vi "Main Interface.vi"() -> ()   [LabVIEW 2013]
panel:
  in  "Current Task":string
  out "Current Progress":u8(slide) scale=0.0..100.0
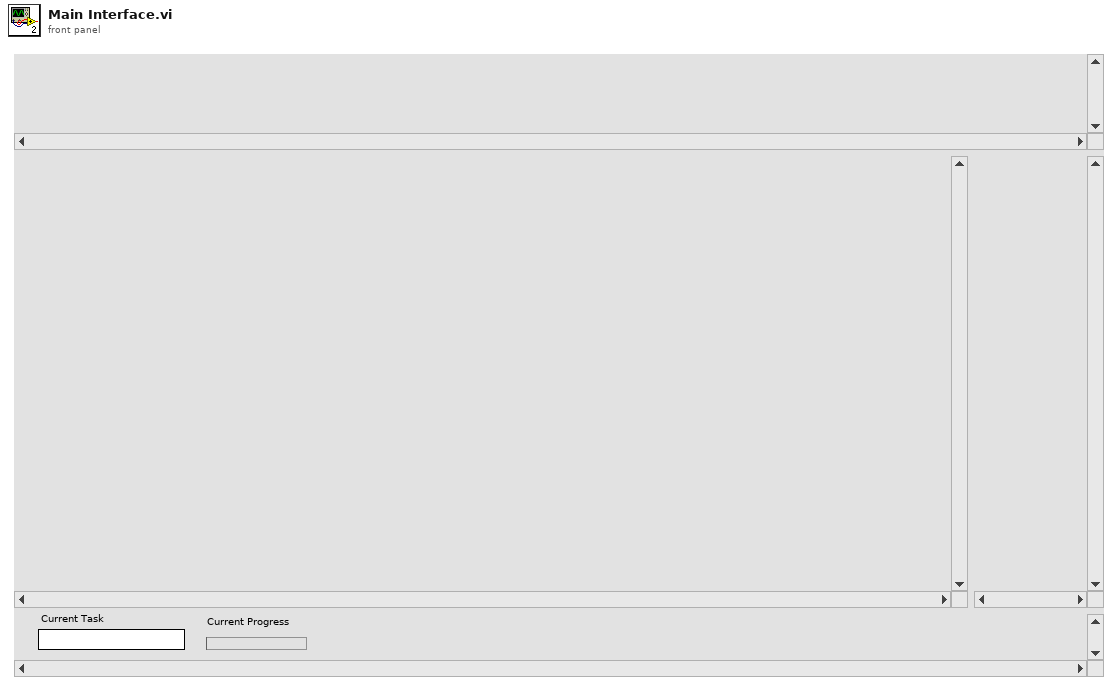
[diagram p1: front panel]
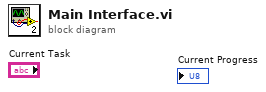
[diagram p0: block diagram]
diagram:
